vi "Ctor.vi"(8 "error in (no error)":errorcluster) -> (0 "error out":errorcluster, 3 "Callback Consumer out":refnum<class "Callback Consumer.lvclass">)   [LabVIEW 2012, in "Callback Consumer.lvclass"]
uses:
  Callback Consumer.lvclass
  Ref Data.ctl
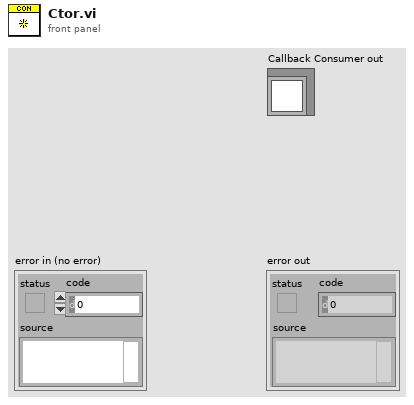
[diagram p1: front panel]
types:
  T1 = typedef "Callback Consumer.lvclass/Ref Data.ctl" = cluster{"Numeric":dbl}
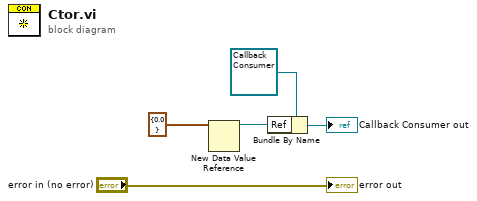
[diagram p0: block diagram]
diagram:
  n1 = New Data Value Reference(data value=T1 {"Numeric"=0.0} ("Ref Data")) -> (data value reference=w1:refnum<data-value>)  [unwired: 1 in, 1 out]
  n2 = Bundle By Name(cluster=refnum<class "Callback Consumer.lvclass"> refnum ("Callback Consumer in"), "Ref"=w1) -> (→"Callback Consumer out":refnum<class "Callback Consumer.lvclass">)
  "error out" <- "error in (no error)"
